vi "LVClass_WavefrontCorrector get all WFC parameter values.vi"(0 "WavefrontCorrector in":refnum<class "WavefrontCorrector.lvclass">, 11 "error in (no error)":errorcluster) -> (4 "WavefrontCorrector out":refnum<class "WavefrontCorrector.lvclass">, 6 "AllWFCParametersValues":T1[](array[typedef]), 15 "error out":errorcluster)   [LabVIEW 2020, in "WavefrontCorrector.lvclass"]
doc: "Description:\nGet current actuators positions.\n\nParameters:\nclass corrector WavefrontCorrector object adress.\nfloat position Array containing the actuators positions.\nError error_in [in] Error\nError error_out [out] Error"
uses:
  WavefrontCorrector.lvclass
  Controls/CameraParametersSetup.ctl
  Controls/CameraParameters_Type.ctl
  WavefrontCorrector.lvclass/WavefrontCorrector.ctl
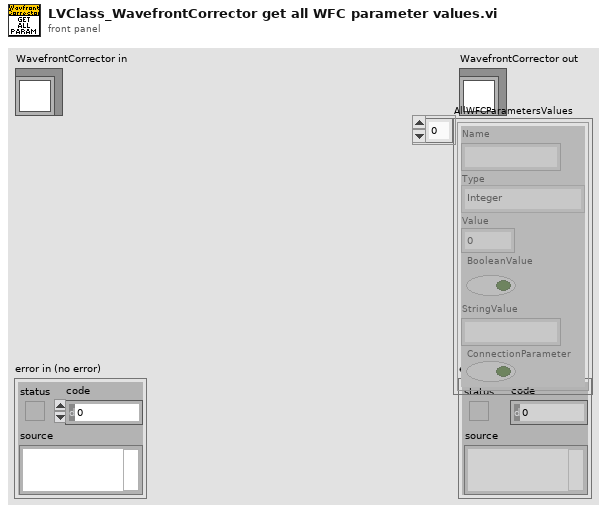
[diagram p1: front panel]
types:
  T1 = typedef "CameraParametersSetup.ctl" = cluster{"Name":string, "Type":T2, "Value":dbl, "BooleanValue":bool, "StringValue":string, "ConnectionParameter":bool}
  T2 = typedef "CameraParameters_Type.ctl" = enum16{"Integer", "Real", "String", "Boolean"}
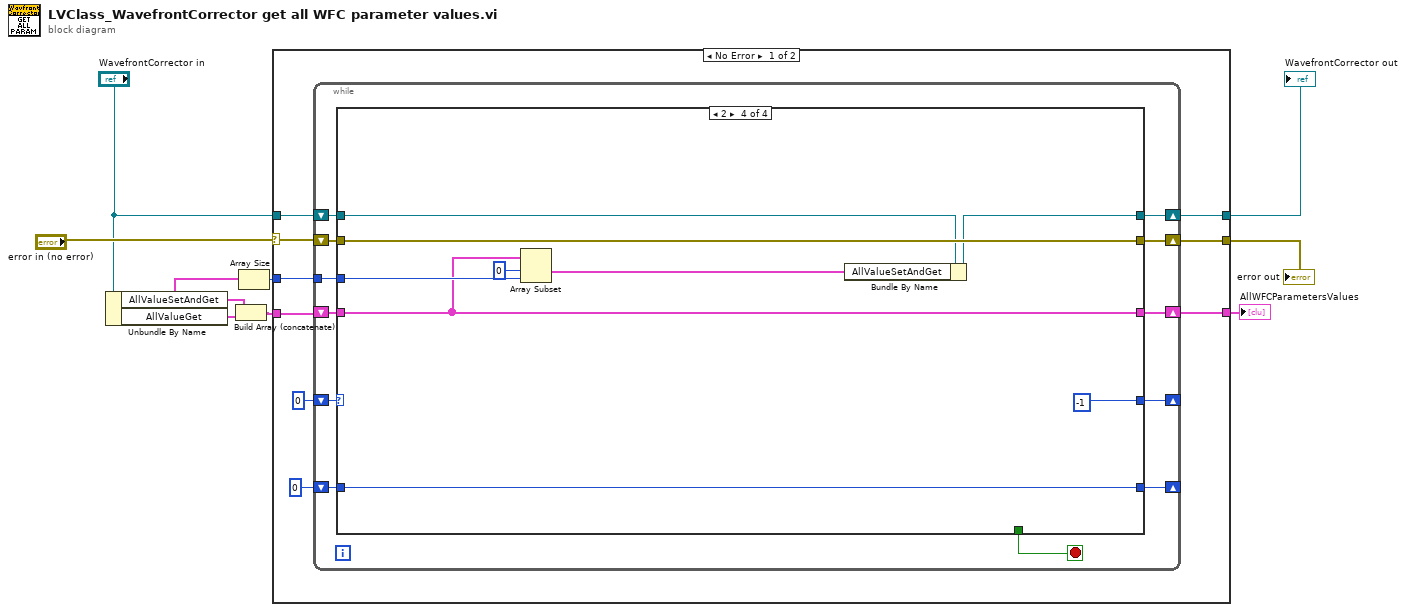
[diagram p0: block diagram]
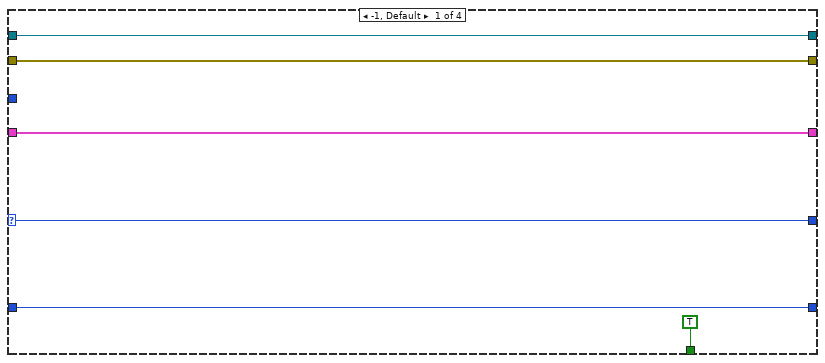
[diagram p2: hidden frame]
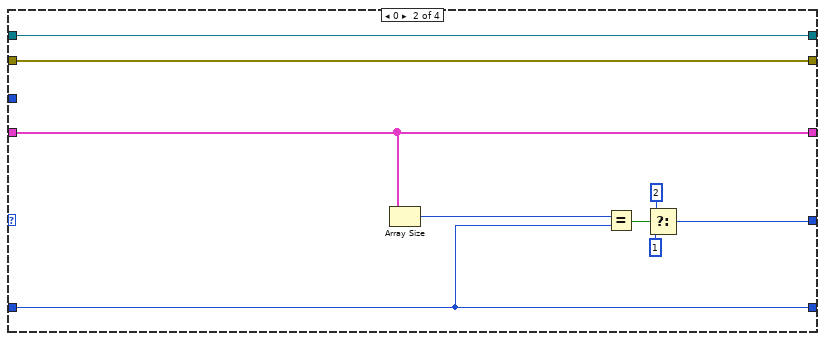
[diagram p3: hidden frame]
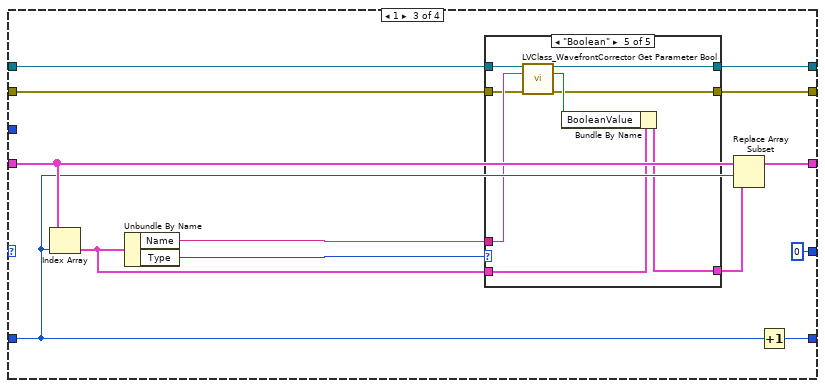
[diagram p4: hidden frame]
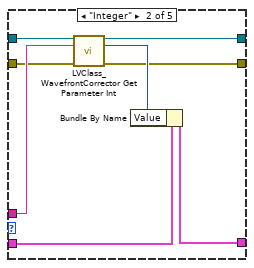
[diagram p6: hidden frame]
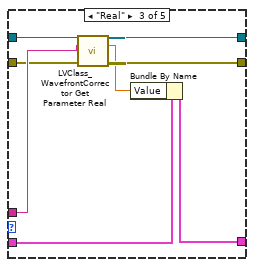
[diagram p7: hidden frame]
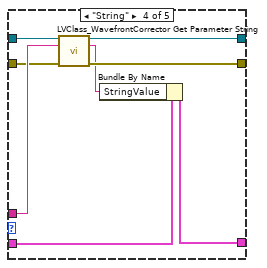
[diagram p8: hidden frame]
diagram:
  n1 = Unbundle By Name("WavefrontCorrector in") -> ("AllValueSetAndGet"=w5:T1[], "AllValueGet"=w4:T1[])
  n2 = Build Array (concatenate)(w5, w4) -> (w2:T1[])
  n3 = Array Size(array=w5) -> (size(s)=w1:i32)
  n4 = case shown="No Error" "error in (no error)" {
    selector: "error in (no error)" -> [w14 w104]
    tunnel: [w15 w104] -> w7
    tunnel: [w16 w103] -> w9
    tunnel: "WavefrontCorrector in" -> [w18 w103]
    tunnel: [w13 _] -> w6
    tunnel: w2 -> [w11 _]
    tunnel: w1 -> [w10 _]
    frame No Error {
      n5 = while {
        shift-right: [w29] -> _
        shift-left: 0 -> [w28]
        shift-right: [w26] -> w15
        shift-left: w14 -> [w25]
        shift-right: [w27] -> w16
        shift-left: w18 -> [w30]
        shift-right: [w23] -> w13
        shift-left: w11 -> [w22]
        shift-right: [w20] -> _
        shift-left: 0 -> [w21]
        tunnel: w10 -> [w19]
        stop <- w24 stop-if-true
        n6 = case shown="2" w28 {
          selector: w28 -> [w33 _ _ _]
          tunnel: w30 -> [w31 w45 w46 w97]
          tunnel: w25 -> [w35 w44 w47 w102]
          tunnel: [w33 w38 0 -1] -> w29
          tunnel: [w31 w45 w57 w96] -> w27
          tunnel: [w35 w44 w56 w102] -> w26
          tunnel: [TRUE _ _ _] -> w24
          tunnel: [w32 w43 w51 w99] -> w23
          tunnel: w22 -> [w32 w43 w53 w99]
          tunnel: w21 -> [w34 w41 w52 w94]
          tunnel: [w34 w41 w55 w94] -> w20
          tunnel: w19 -> [_ _ _ w100]
          frame -1, Default {
          }
          frame 0 {
            n7 = Array Size(array=w43) -> (size(s)=w42:i32)
            n8 = Equal?(x=w42, y=w41) -> (x = y?=w40:bool)
            n9 = Select(t=2, s=w40, f=1) -> (s? t:f=w38:i32)
          }
          frame 1 {
            n10 = Index Array(array=w53, index=w52) -> (element=w54:T1)
            n11 = Unbundle By Name(w54) -> ("Name"=w49:string, "Type"=w50:T2)
            n12 = case shown="\"Boolean\"" w50 {
              tunnel: w54 -> [w59 w69 w70 w78 w87]
              tunnel: [w59 w68 w71 w85 w86] -> w48
              tunnel: w49 -> [_ w67 w76 w82 w92]
              tunnel: w46 -> [w61 w66 w77 w84 w93]
              tunnel: [w61 w65 w73 w83 w90] -> w57
              tunnel: [w60 w63 w74 w80 w88] -> w56
              tunnel: w47 -> [w60 w62 w75 w81 w91]
              frame Default {
              }
              frame "Integer" {
                n13 = call "LVClass_WavefrontCorrector Get Parameter Int.vi"("WavefrontCorrector in"=w66, "parameter_name"=w67, "error in (no error)"=w62) -> ("WavefrontCorrector out"=w65:refnum<class "WavefrontCorrector.lvclass">, "value"=w64:i32, "error out"=w63:errorcluster)  [unwired: 10 in]
                n14 = Bundle By Name(cluster=w69, "Value"=w64) -> (w68:T1)
              }
              frame "Real" {
                n15 = call "LVClass_WavefrontCorrector Get Parameter Real.vi"("WavefrontCorrector in"=w77, "parameter_name"=w76, "error in (no error)"=w75) -> ("WavefrontCorrector out"=w73:refnum<class "WavefrontCorrector.lvclass">, "value"=w72:dbl, "error out"=w74:errorcluster)  [unwired: 10 in]
                n16 = Bundle By Name(cluster=w70, "Value"=w72) -> (w71:T1)
              }
              frame "String" {
                n17 = call "LVClass_WavefrontCorrector Get Parameter String.vi"("WavefrontCorrector in"=w84, "parameter_name"=w82, "error in (no error)"=w81) -> ("WavefrontCorrector out"=w83:refnum<class "WavefrontCorrector.lvclass">, "value"=w79:string, "error out"=w80:errorcluster)  [unwired: 10 in]
                n18 = Bundle By Name(cluster=w78, "StringValue"=w79) -> (w85:T1)
              }
              frame "Boolean" {
                n19 = call "LVClass_WavefrontCorrector Get Parameter Bool.vi"("WavefrontCorrector in"=w93, "parameter_name"=w92, "error in (no error)"=w91) -> ("WavefrontCorrector out"=w90:refnum<class "WavefrontCorrector.lvclass">, "value"=w89:bool, "error out"=w88:errorcluster)  [unwired: 10 in]
                n20 = Bundle By Name(cluster=w87, "BooleanValue"=w89) -> (w86:T1)
              }
            }
            n21 = Replace Array Subset(array=w53, new element=w48, index=w52) -> (w51:T1[])
            n22 = Increment(x=w52) -> (x+1=w55:i32)
          }
          frame 2 {
            n23 = Array Subset(array=w99, index=0, length=w100) -> (w98:T1[])
            n24 = Bundle By Name(cluster=w97, "AllValueSetAndGet"=w98) -> (w96:refnum<class "WavefrontCorrector.lvclass">)
          }
        }
      }
    }
    frame Error {
    }
  }
  "error out" <- w7
  "WavefrontCorrector out" <- w9
  "AllWFCParametersValues" <- w6
